vi "机柜空调告警状态解析.vi"(11 "输入字符串":string) -> (3 "机柜空调告警状态":T1)   [LabVIEW 2016, in "环境动力监测库.lvlib" / "空调库.lvlib"]
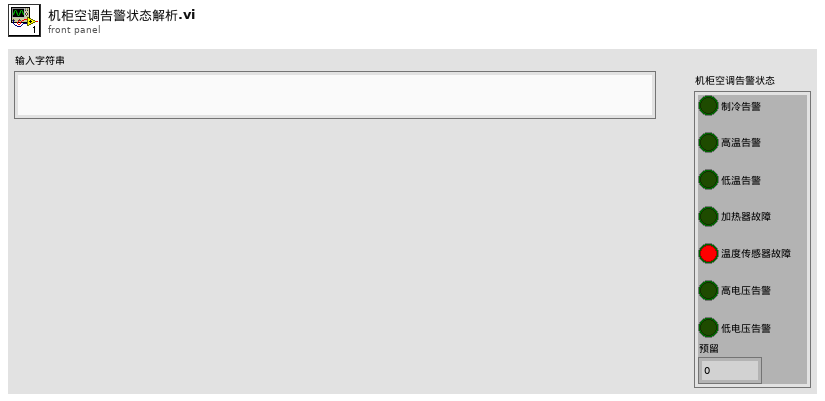
[diagram p1: front panel]
types:
  T1 = cluster{"制冷告警":bool, "高温告警":bool, "低温告警":bool, "加热器故障":bool, "温度传感器故障":bool, "高电压告警":bool, "低电压告警":bool, "预留":u16}
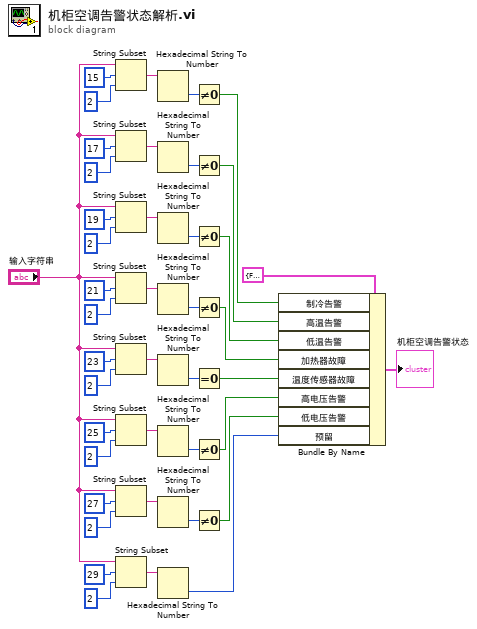
[diagram p0: block diagram]
diagram:
  n1 = String Subset(string="输入字符串", offset (0)=15 ("偏移量(0)"), length (rest)=2 ("长度（剩余）")) -> (substring=w40:string)
  n2 = String Subset(string="输入字符串", offset (0)=17 ("偏移量(0)"), length (rest)=2 ("长度（剩余）")) -> (substring=w37:string)
  n3 = String Subset(string="输入字符串", offset (0)=19 ("偏移量(0)"), length (rest)=2 ("长度（剩余）")) -> (substring=w36:string)
  n4 = String Subset(string="输入字符串", offset (0)=21 ("偏移量(0)"), length (rest)=2 ("长度（剩余）")) -> (substring=w31:string)
  n5 = String Subset(string="输入字符串", offset (0)=23 ("偏移量(0)"), length (rest)=2 ("长度（剩余）")) -> (substring=w21:string)
  n6 = String Subset(string="输入字符串", offset (0)=25 ("偏移量(0)"), length (rest)=2 ("长度（剩余）")) -> (substring=w24:string)
  n7 = String Subset(string="输入字符串", offset (0)=27 ("偏移量(0)"), length (rest)=2 ("长度（剩余）")) -> (substring=w25:string)
  n8 = String Subset(string="输入字符串", offset (0)=29 ("偏移量(0)"), length (rest)=2 ("长度（剩余）")) -> (substring=w30:string)
  n9 = Hexadecimal String To Number(string=w40) -> (number=w17:u32)  [unwired: 2 in, 1 out]
  n10 = Hexadecimal String To Number(string=w37) -> (number=w14:u32)  [unwired: 2 in, 1 out]
  n11 = Hexadecimal String To Number(string=w36) -> (number=w12:u32)  [unwired: 2 in, 1 out]
  n12 = Hexadecimal String To Number(string=w31) -> (number=w10:u32)  [unwired: 2 in, 1 out]
  n13 = Hexadecimal String To Number(string=w21) -> (number=w8:u32)  [unwired: 2 in, 1 out]
  n14 = Hexadecimal String To Number(string=w24) -> (number=w6:u32)  [unwired: 2 in, 1 out]
  n15 = Hexadecimal String To Number(string=w25) -> (number=w4:u32)  [unwired: 2 in, 1 out]
  n16 = Hexadecimal String To Number(string=w30) -> (number=w2:u32)  [unwired: 2 in, 1 out]
  n17 = Not Equal To 0?(x=w17) -> (x != 0?=w15:bool)
  n18 = Not Equal To 0?(x=w14) -> (x != 0?=w13:bool)
  n19 = Not Equal To 0?(x=w12) -> (x != 0?=w11:bool)
  n20 = Not Equal To 0?(x=w10) -> (x != 0?=w9:bool)
  n21 = Equal To 0?(x=w8) -> (x = 0?=w7:bool)
  n22 = Not Equal To 0?(x=w6) -> (x != 0?=w5:bool)
  n23 = Not Equal To 0?(x=w4) -> (x != 0?=w3:bool)
  n24 = Bundle By Name(cluster=T1 {"制冷告警"=FALSE, "高温告警"=FALSE, "低温告警"=FALSE, "加热器故障"=FALSE, "温度传感器故障"=FALSE, "高电压告警"=FALSE, "低电压告警"=FALSE, "预留"=0} ("机柜空调告警状态 2"), "制冷告警"=w15, "高温告警"=w13, "低温告警"=w11, "加热器故障"=w9, "温度传感器故障"=w7, "高电压告警"=w5, "低电压告警"=w3, "预留"=w2) -> (→"机柜空调告警状态":T1)
